vi "Add Tests.vi"(10 "Tests":string[](array[string]), 11 "Result Model In":refnum<class "Result Model.lvclass">) -> (3 "Result Model Out":refnum<class "Result Model.lvclass">)   [LabVIEW 2020, in "Result Model.lvclass"]
uses:
  Result Model.lvclass
  Result Model.lvclass/Result Model.ctl
  Result/Status.ctl
  Result/Result.lvlib
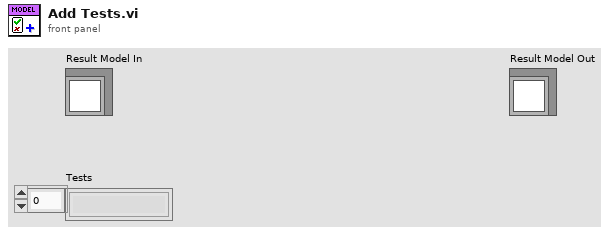
[diagram p1: front panel]
types:
  T1 = typedef "Result.lvlib/Status.ctl" = enum16{"", "Passed", "Failed", "Error", "Skipped", "Setup Error", "Broken", "Teardown Error"}
  T2 = typedef "Result Model.lvclass/Model State.ctl" = cluster{"Run Queue":set{string}, "Test Statuses":map{string, T1}, "Execution Time":map{string, dbl}, "Assertions":map{string, cluster{"Result Type":T3, "Status":T1, "Message":string, "Description":string}[]}}
  T3 = typedef "Result.lvlib/Type.ctl" = enum16{"Method", "Case", "Suite", "Pass", "Fail", "Skip", "Pass if", "Fail if", "Pass if Error", "Fail if Error", "Pass if Equal", "Fail if Equal"}
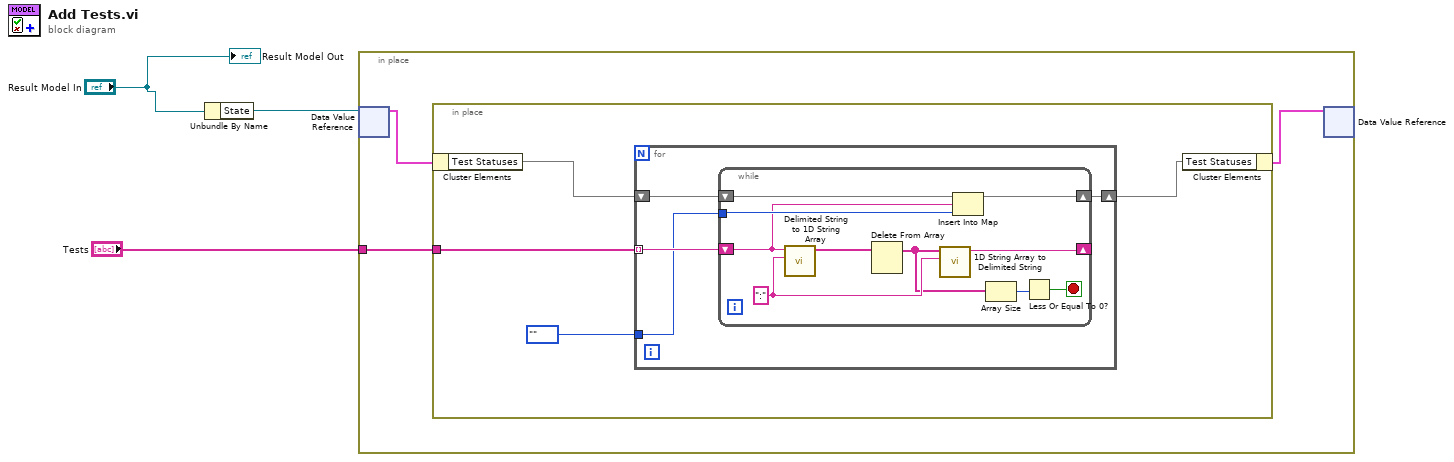
[diagram p0: block diagram]
diagram:
  n1 = Unbundle By Name("Result Model In") -> ("State"=w2:refnum<data-value>)
  n2 = in-place {
    in-place-border: "Tests" -> [w6]
    n3 = in-place-dvr #1(w2) -> (w5:T2)  [unwired: 1 out]
    n4 = in-place {
      in-place-border: w6 -> [w10]
      n5 = in-place-cluster #2(w5) -> ("Test Statuses"=w8:map{string, T1})
      n6 = for {
        tunnel: w10 -> [w12] mode=indexing
        shift-right: [w13] -> w7
        shift-left: w8 -> [w14]
        tunnel: Status."" ("Status") -> [w11]
        n7 = while {
          tunnel: w11 -> [w22]
          shift-right: [w23] -> w13
          shift-left: w14 -> [w24]
          shift-right: [w17] -> _
          shift-left: w12 -> [w20]
          stop <- w15 stop-if-true
          w19 = ":" ("delimiter")
          n8 = call <vilib>:"Delimited String to 1D String Array.vi"("delimiter"=w19, "delimited string"=w20) -> ("string array"=w21:string[])  [unwired: 9 in]
          n9 = Delete From Array(array=w21) -> (array with subset deleted=w18:string[])  [unwired: 2 in, 1 out]
          n10 = call <vilib>:"1D String Array to Delimited String.vi"("delimiter"=w19, "string array"=w18) -> ("delimited string"=w17:string)  [unwired: 9 in]
          n11 = Insert Into Map(map in=w24, key=w20, value=w22) -> (map out=w23:map{string, T1})  [unwired: 2 out]
          n12 = Array Size(array=w18) -> (size(s)=w16:i32)
          n13 = Less Or Equal To 0?(x=w16) -> (x <= 0?=w15:bool)
        }
      }
      n14 = in-place-cluster #2("Test Statuses"=w7) -> (w4:T2)
    }
    n15 = in-place-dvr #1(w4) -> ()  [unwired: 2 out]
  }
  "Result Model Out" <- "Result Model In"
